vi "Generate Text Report.vi"(8 "error in (no error)":errorcluster, 11 "Plain Text Report In":refnum<class "Plain Text Report.lvclass">) -> (0 "error out":errorcluster, 2 "Text":string, 3 "Plain Text Report Out":refnum<class "Plain Text Report.lvclass">)   [LabVIEW 2020, in "Plain Text Report.lvclass"]
uses:
  Plain Text Report.lvclass
  C:/git/astemes-lunit/source/Framework/Report Classes/Test Report/Test Report.lvclass
  Plain Text Report.lvclass/Plain Text Report.ctl
  Test Report/Test Report.lvclass/Test Report.ctl
  Test Report/Test Report.lvclass
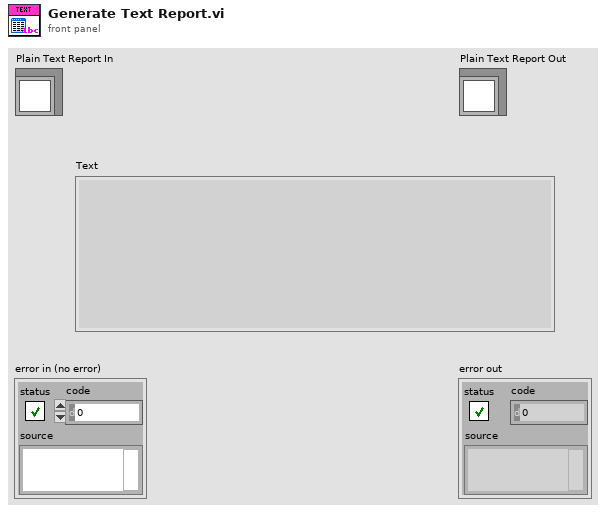
[diagram p1: front panel]
types:
  T1 = typedef "Test Suite Result.lvlib/Test Suite Result.ctl" = cluster{"Test Suite ID":string, "Name":string, "Hostname":string, "Status":T2, "Execution time":dbl, "Start Time":timestamp, "Case Results":T3[]}
  T2 = typedef "Result.lvlib/Status.ctl" = enum16{"", "Passed", "Failed", "Error", "Skipped", "Setup Error", "Broken", "Teardown Error"}
  T3 = typedef "Test Case Result.lvlib/Test Case Result.ctl" = map{string, T4}
  T4 = typedef "Method Result.lvlib/Method Result.ctl" = cluster{"Test Case":string, "Test Method Name":string, "Status":T2, "Assertion Results":T5[], "Execution time":dbl, "Result String":string}
  T5 = typedef "Assertion Result.lvlib/Assertion Result.ctl" = cluster{"Status":T2, "Message":string, "Description":string, "Assertion Type":T6}
  T6 = typedef "Result.lvlib/Assertion Type.ctl" = enum16{"None", "Pass", "Fail", "Skip", "Pass if Equal", "Fail if Equal", "Pass if Error", "Fail if Error", "Pass if", "Fail if"}
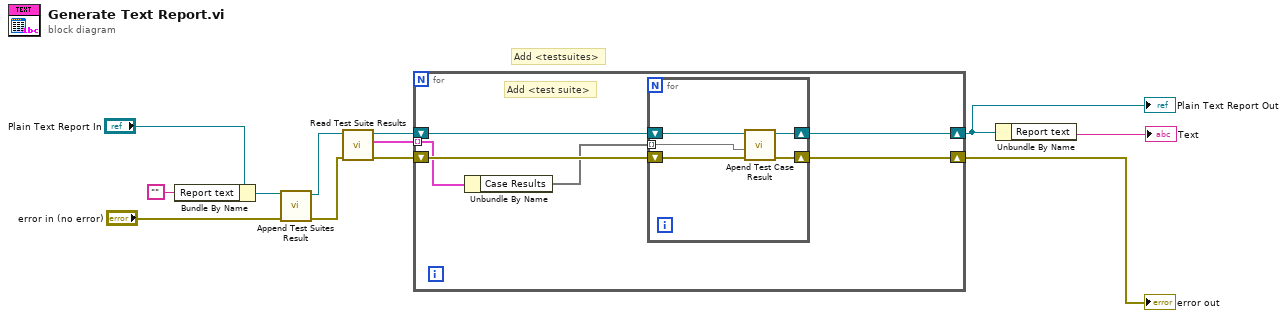
[diagram p0: block diagram]
diagram:
  # "Add <testsuites>"
  n1 = Bundle By Name(cluster="Plain Text Report In", "Report text"="") -> (w2:refnum<class "Plain Text Report.lvclass">)
  n2 = call "Append Test Suites Result.vi"("error in (no error)"="error in (no error)", "Plain Text Report In"=w2) -> ("error out"=w7:errorcluster, "Plain Text Report Out"=w9:refnum<class "Plain Text Report.lvclass">)  [unwired: 8 in]
  n3 = call "Read Test Suite Results.vi"("error in (no error)"=w7, "Report In"=w9) -> ("error out"=w6:errorcluster, "Test Suite Results"=w10:T1[], "Report Out"=w8:refnum<class "Plain Text Report.lvclass">)  [unwired: 7 in]
  n4 = for {
    tunnel: w10 -> [w14] mode=indexing
    shift-right: [w17] -> w5
    shift-left: w6 -> [w15]
    shift-right: [w16] -> w4
    shift-left: w8 -> [w18]
    # "Add <test suite>"
    n5 = Unbundle By Name(w14) -> ("Case Results"=w13:T3[])
    n6 = for {
      tunnel: w13 -> [w22] mode=indexing
      shift-right: [w20] -> w17
      shift-left: w15 -> [w23]
      shift-right: [w19] -> w16
      shift-left: w18 -> [w21]
      n7 = call "Apend Test Case Result.vi"("error in (no error)"=w23, "Test Case Result"=w22, "Plain Text Report In"=w21) -> ("error out"=w20:errorcluster, "Plain Text Report Out"=w19:refnum<class "Plain Text Report.lvclass">)  [unwired: 7 in]
    }
  }
  "error out" <- w5
  "Plain Text Report Out" <- w4
  n8 = Unbundle By Name(w4) -> ("Report text"=→"Text":string)
